vi "AutoPlayParser.vi"(0 "Auto Play":string) -> (1 "Drive Mode Strings":string[](array[string]), 2 "Drive Command Strings":string[](array[string]), 3 "Subsystem VI References":path[](array[path]), 4 "Subsystem Command Strings":string[](array[string]))   [LabVIEW 2019]
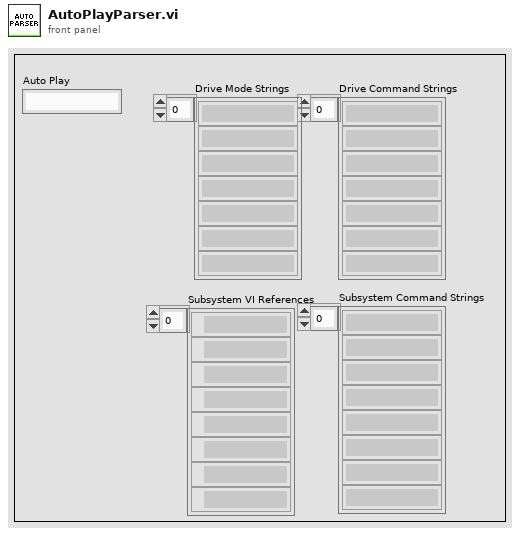
[diagram p1: front panel]
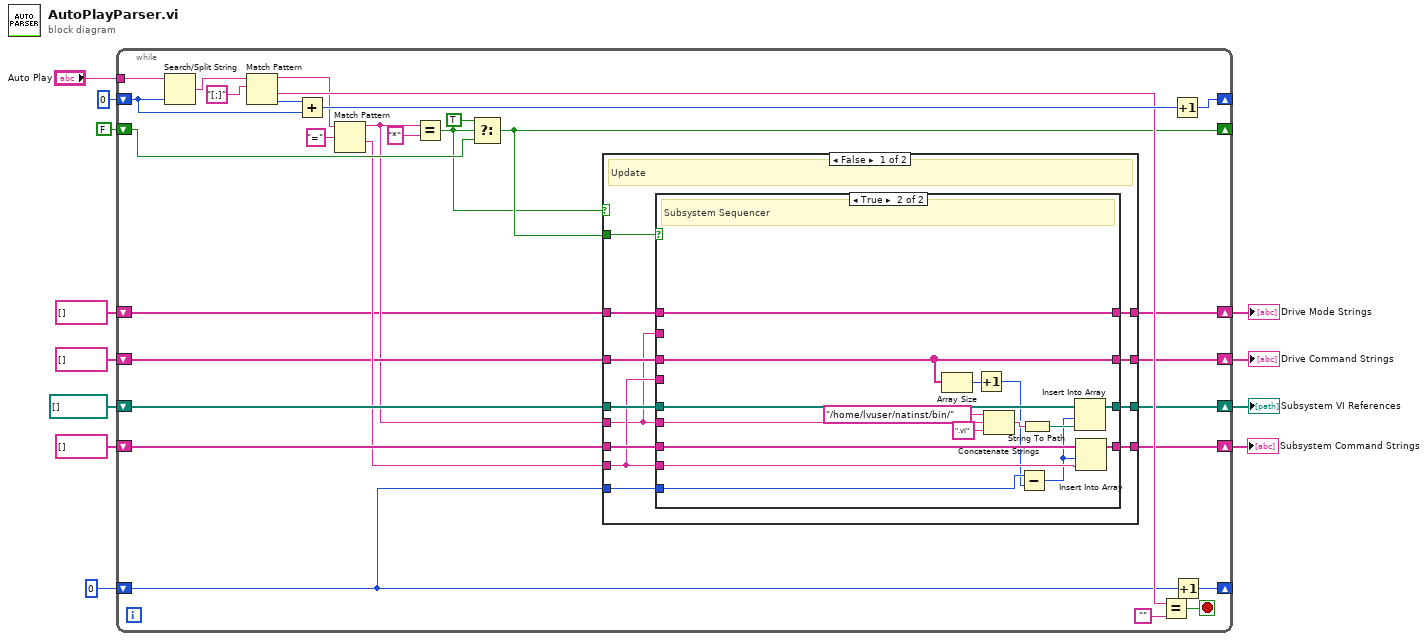
[diagram p0: block diagram]
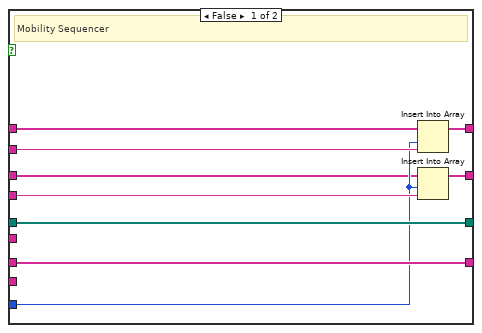
[diagram p2: hidden frame]
diagram:
  n1 = while {
    tunnel: "Auto Play" -> [w38]
    shift-right: [w33] -> _
    shift-left: 0 ("offset (0)") -> [w35]
    shift-right: [w29] -> _
    shift-left: 0 -> [w21]
    shift-right: [w28] -> w10
    shift-left: path[] [] -> [w27]
    shift-right: [w26] -> w9
    shift-left: string[] [] -> [w25]
    shift-right: [w20] -> _
    shift-left: FALSE -> [w22]
    shift-right: [w18] -> w7
    shift-left: string[] [] -> [w17]
    shift-right: [w15] -> w6
    shift-left: string[] [] -> [w14]
    stop <- w40 stop-if-true
    n2 = Search/Split String(string=w38, offset (0)=w35) -> (match + rest of string=w37:string)  [unwired: 1 in, 2 out]
    n3 = Match Pattern(string=w37, regular expression="[;]") -> (before substring=w30:string, after substring=w32:string, offset past match=w36:i32)  [unwired: 1 in, 1 out]
    n4 = Add(x=w36, y=w35) -> (x+y=w34:i32)
    n5 = Match Pattern(string=w30, regular expression="=") -> (before substring=w16:string, after substring=w19:string)  [unwired: 1 in, 2 out]
    n6 = Equal?(x=w16, y="*") -> (x = y?=w13:bool)
    n7 = Select(t=TRUE, s=w13, f=w22) -> (s? t:f=w20:bool)
    n8 = case shown="False" w13 {
      tunnel: [w53 w80] -> w28
      tunnel: w27 -> [w52 w80]
      tunnel: [w51 w79] -> w26
      tunnel: w25 -> [w50 w79]
      tunnel: w21 -> [w49 _]
      tunnel: w20 -> [w48 _]
      tunnel: w19 -> [w47 _]
      tunnel: [w46 w81] -> w18
      tunnel: w17 -> [w45 w81]
      tunnel: w16 -> [w44 _]
      tunnel: [w43 w82] -> w15
      tunnel: w14 -> [w42 w82]
      frame False {
        # "Update"
        n9 = case shown="True" w48 {
          tunnel: [w62 w77] -> w53
          tunnel: w52 -> [w62 w76]
          tunnel: w47 -> [_ w75]
          tunnel: [w61 w74] -> w51
          tunnel: w50 -> [w61 w73]
          tunnel: w44 -> [_ w70]
          tunnel: w49 -> [w55 w67]
          tunnel: w47 -> [w60 _]
          tunnel: [w59 w68] -> w46
          tunnel: w45 -> [w54 w68]
          tunnel: w44 -> [w58 _]
          tunnel: [w57 w69] -> w43
          tunnel: w42 -> [w56 w69]
          frame False {
            # "Mobility Sequencer"
            n10 = Insert Into Array(array=w56, index=w55, new element=w58) -> (w57:string[])
            n11 = Insert Into Array(array=w54, index=w55, new element=w60) -> (w59:string[])
          }
          frame True {
            # "Subsystem Sequencer"
            n12 = Array Size(array=w68) -> (size(s)=w66:i32)
            n13 = Increment(x=w66) -> (x+1=w64:i32)
            n14 = Concatenate Strings("/home/lvuser/natinst/bin/" ("string"), w70, ".vi" ("string")) -> (w71:string)
            n15 = Subtract(x=w67, y=w64) -> (x-y=w65:i32)
            n16 = String To Path(string=w71) -> (path=w78:path)
            n17 = Insert Into Array(array=w76, index=w65, new element=w78) -> (w77:path[])
            n18 = Insert Into Array(array=w73, index=w65, new element=w75) -> (w74:string[])
          }
        }
      }
      frame True {
        # "Skip Break Line"
      }
    }
    n19 = Equal?(x=w32, y="") -> (x = y?=w40:bool)
    n20 = Increment(x=w34) -> (x+1=w33:i32)
    n21 = Increment(x=w21) -> (x+1=w29:i32)
  }
  "Subsystem VI References" <- w10
  "Subsystem Command Strings" <- w9
  "Drive Command Strings" <- w7
  "Drive Mode Strings" <- w6
